vi "data_to_xml.vi"(8 "error in (no error)":errorcluster, 11 "Counter in":refnum<class "Counter.lvclass">) -> (0 "error out":errorcluster, 2 "counter data string":string, 3 "Counter out":refnum<class "Counter.lvclass">)   [LabVIEW 2013, in "Counter.lvclass"]
uses:
  Counter.lvclass
  Counter.lvclass/Counter.ctl
  Experiment/Globals.vi
  TCP_IP/TCP_IP.lvclass
  Experiment/Experiment.lvclass
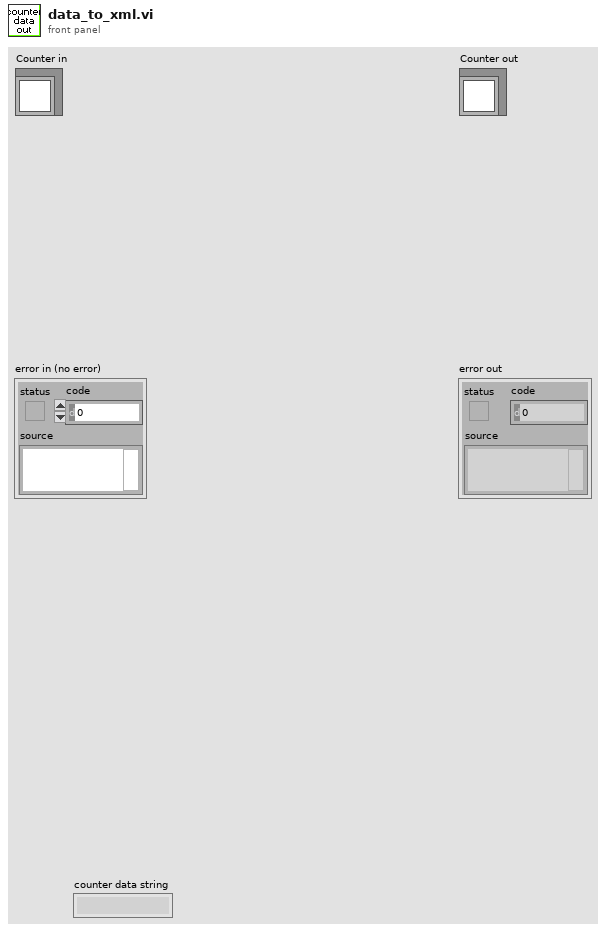
[diagram p1: front panel]
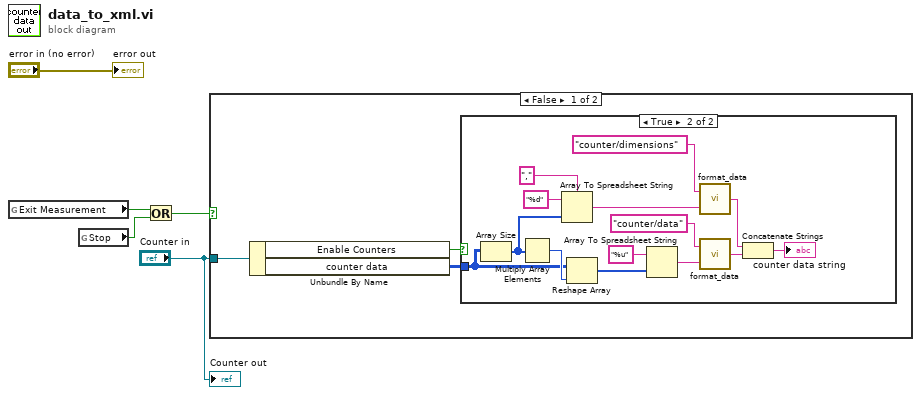
[diagram p0: block diagram]
diagram:
  n1 = global read "Globals.vi" "Exit Measurement"() -> (w3:bool)
  n2 = global read "Globals.vi" "Stop"() -> (w2:bool)
  n3 = Or(x=w3, y=w2) -> (x .or. y?=w1:bool)
  n4 = case shown="False" w1 {
    tunnel: "Counter in" -> [w8 _]
    frame False {
      n5 = Unbundle By Name(w8) -> ("Enable Counters"=w6:bool, "counter data"=w7:u32[][])
      n6 = case shown="True" w6 {
        tunnel: w7 -> [_ w20]
        frame False {
        }
        frame True {
          n7 = Array Size(array=w20) -> (size(s)=w16:i32[])
          n8 = Multiply Array Elements(1:w16) -> (0:w21:i32)
          n9 = Array To Spreadsheet String(delimiter (Tab)=",", array=w16, 3:"%d" ("format string")) -> (spreadsheet string=w14:string)
          n10 = Reshape Array(w20, w21) -> (w19:u32[])
          n11 = Array To Spreadsheet String(array=w19, 3:"%u" ("format string")) -> (spreadsheet string=w12:string)  [unwired: 1 in]
          n12 = call "format_data.vi"("data"=w14, "name"="counter/dimensions") -> ("concatenated string"=w11:string)
          n13 = call "format_data.vi"("data"=w12, "name"="counter/data") -> ("concatenated string"=w10:string)
          n14 = Concatenate Strings(w11, w10) -> (→"counter data string":string)
        }
      }
    }
    frame True {
    }
  }
  "error out" <- "error in (no error)"
  "Counter out" <- "Counter in"
